vi "EnqueueManager__slk_QSM-PC (String).vi"   [LabVIEW 2009, in "QSM-PC (String).lvlib"]
doc: "Sets elements to the different position of queue.\n\n<b>Functions:</b>\nEnqueue to the back of queue\nEnqueue to the front of queue\nReplace the elements of queue"
uses:
  Library/QSM-PC (String).lvlib
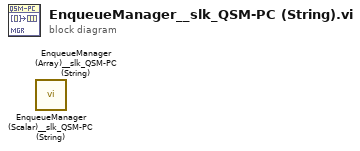
[diagram p0: block diagram]
diagram:
  n1 = call "EnqueueManager (Scalar)__slk_QSM-PC (String).vi"() -> ()  [unwired: 11 in, 1 out]
  n2 = call "EnqueueManager (Array)__slk_QSM-PC (String).vi"() -> ()  [unwired: 11 in, 1 out]
